vi "Init from Tick Count.vi"(8 "error in":errorcluster, 10 "Tick Count (ms)":u64, 11 "Timestamp in":refnum<class "Timestamp.lvclass">) -> (0 "error out":errorcluster, 3 "Time Stamp out":refnum<class "Timestamp.lvclass">)   [LabVIEW 2024, in "Timestamp.lvclass"]
uses:
  Timestamp.lvclass
  Timestamp.lvclass/Timestamp.ctl
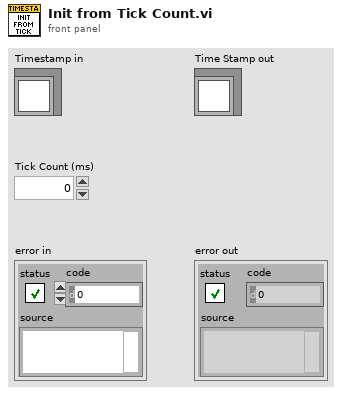
[diagram p1: front panel]
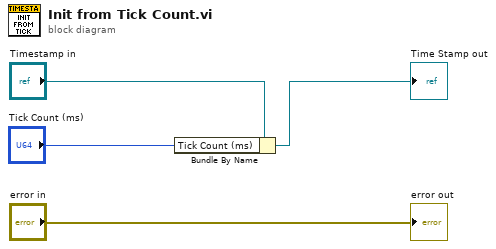
[diagram p0: block diagram]
diagram:
  n1 = Bundle By Name(cluster="Timestamp in", "Tick Count (ms)"="Tick Count (ms)") -> (→"Time Stamp out":refnum<class "Timestamp.lvclass">)
  "error out" <- "error in"
